vi "Test6.vi"() -> ()   [LabVIEW 2010]
uses:
  <vilib>/MDSplus/Classes/Tree_Class/Tree.lvclass
  <vilib>/MDSplus/Classes/Data_Class/Scalar_Class/Float32_Class/Float32.lvclass
  <vilib>/MDSplus/Classes/Data_Class/Data.lvclass
  <vilib>/MDSplus/Classes/Data_Class/TreeNode_Class/TreeNode.lvclass
panel:
  in  "Value":sgl=6.666
  in  "Path":string=":NUMX"
  in  "Mode":string="EDIT"
  in  "Shot":i32=-1
  in  "Name":string="my_tree"
  out "Float out":sgl
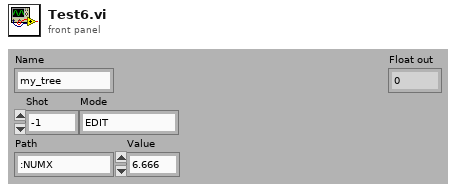
[diagram p1: front panel]
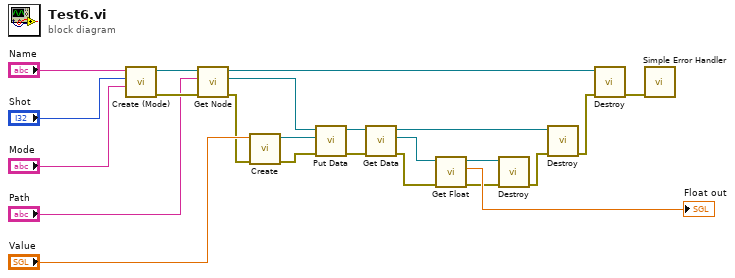
[diagram p0: block diagram]
diagram:
  n1 = call <vilib>:"Create (Mode).vi"("Mode"="Mode", "Shot"="Shot", "Name"="Name") -> ("error out"=w19:errorcluster, "Tree out"=w20:refnum<class "Tree.lvclass">)  [unwired: 7 in]
  n2 = call-dynamic "Get Node.vi"("error in (no error)"=w19, "Path"="Path", "Tree in"=w20) -> ("error out"=w2:errorcluster, "Node out"=w16:refnum<class "TreeNode.lvclass">, "Tree out"=w7:refnum<class "Tree.lvclass">)  [unwired: 6 in]
  n3 = call <vilib>:"Create.vi"("error in (no error)"=w2, "SGL in"="Value") -> ("error out"=w1:errorcluster, "Float32 out"=w6:refnum<class "Float32.lvclass">)  [unwired: 8 in]
  n4 = call-dynamic "Put Data.vi"("error in (no error)"=w1, "Data in"=w6, "TreeNode in"=w16) -> ("error out"=w3:errorcluster, "TreeNode out"=w4:refnum<class "TreeNode.lvclass">)  [unwired: 6 in, 1 out]
  n5 = call-dynamic "Get Data.vi"("error in (no error)"=w3, "TreeNode in"=w4) -> ("error out"=w14:errorcluster, "Data out"=w15:refnum<class "Data.lvclass">, "TreeNode out"=w9:refnum<class "TreeNode.lvclass">)  [unwired: 7 in]
  n6 = call-dynamic "Get Float.vi"("error in (no error)"=w14, "Data in"=w15) -> ("error out"=w11:errorcluster, "SGL out"=→"Float out":sgl, "Data out"=w13:refnum<class "Data.lvclass">)  [unwired: 7 in]
  n7 = call-dynamic "Destroy.vi"("error in (no error)"=w11, "Data in"=w13) -> ("error out"=w8:errorcluster)  [unwired: 9 in]
  n8 = call-dynamic "Destroy.vi"("error in (no error)"=w8, "TreeNode in"=w9) -> ("error out"=w10:errorcluster)  [unwired: 9 in]
  n9 = call-dynamic "Destroy.vi"("error in (no error)"=w10, "Tree in"=w7) -> ("error out"=w5:errorcluster)  [unwired: 8 in]
  n10 = call <vilib>:"Simple Error Handler.vi"("error in (no error)"=w5) -> ()  [unwired: 4 in, 5 out]
